vi "Image Flatfield Correction (SGL).vi"(8 "error in (no error)":errorcluster, 10 "Flatfield Correction":T2={"Flatfield Estimation Options"={"Sampling Grid Size X"=0, "Sampling Grid Size Y"=256, "Polynomial Degree"=0}, "Background Options"={"Estimate Background"=FALSE, "Background Estimation Size"=0, "Niblack Deviation Factor [0. 1]"=0.0}, "Correction Factor"=0.0}, 11 "Refnum in":T1) -> (0 "error out":errorcluster, 3 "Refnum out":T1)   [LabVIEW 2021, in "Image.lvlib"]
uses:
  Image.lvlib
  Flatfield Correction Options.ctl
  <vilib>/vision/Image Controls.llb/IMAQ Image.ctl
  <vilib>/vision/Process.llb/Surface Fit Options.ctl
  <vilib>/vision/Process.llb/Background Estimation Options.ctl
  <vilib>/vision/NI_Vision_Development_Module.lvlib
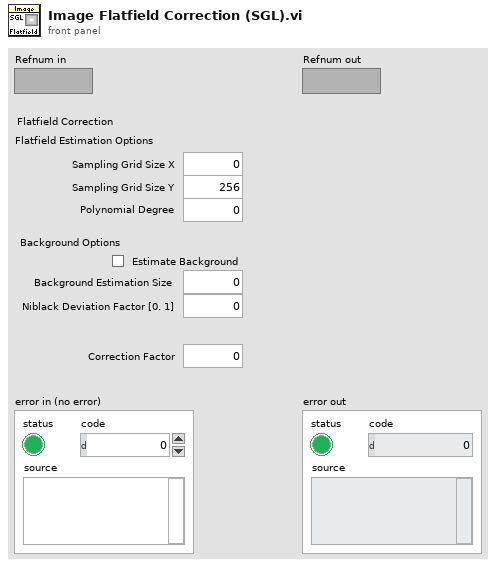
[diagram p1: front panel]
types:
  T1 = typedef "IMAQ Image.ctl" = refnum<image>
  T2 = typedef "Image.lvlib/Flatfield Correction Options.ctl" = cluster{"Flatfield Estimation Options":cluster{"Sampling Grid Size X":i32, "Sampling Grid Size Y":i32, "Polynomial Degree":i32}, "Background Options":cluster{"Estimate Background":bool, "Background Estimation Size":i32, "Niblack Deviation Factor [0. 1]":dbl}, "Correction Factor":sgl}
  T3 = typedef "Background Estimation Options.ctl" = cluster{"Estimate Background?":bool, "Method":i32, "Polynomial Degree":i32, "Window Size (32x32)":cluster{"SizeX":i32, "SizeY":i32}, "Niblack Deviation Factor (0.2)":dbl}
  T4 = cluster{"Line Scan Image?":bool, "Correction Factor":sgl}
  T5 = typedef "Surface Fit Options.ctl" = cluster{"Model":i32, "Sampling Grid Size":cluster{"SizeX":i32, "SizeY":i32}, "Polynomial Degree":i32}
  T6 = typedef "Image Type" = u32
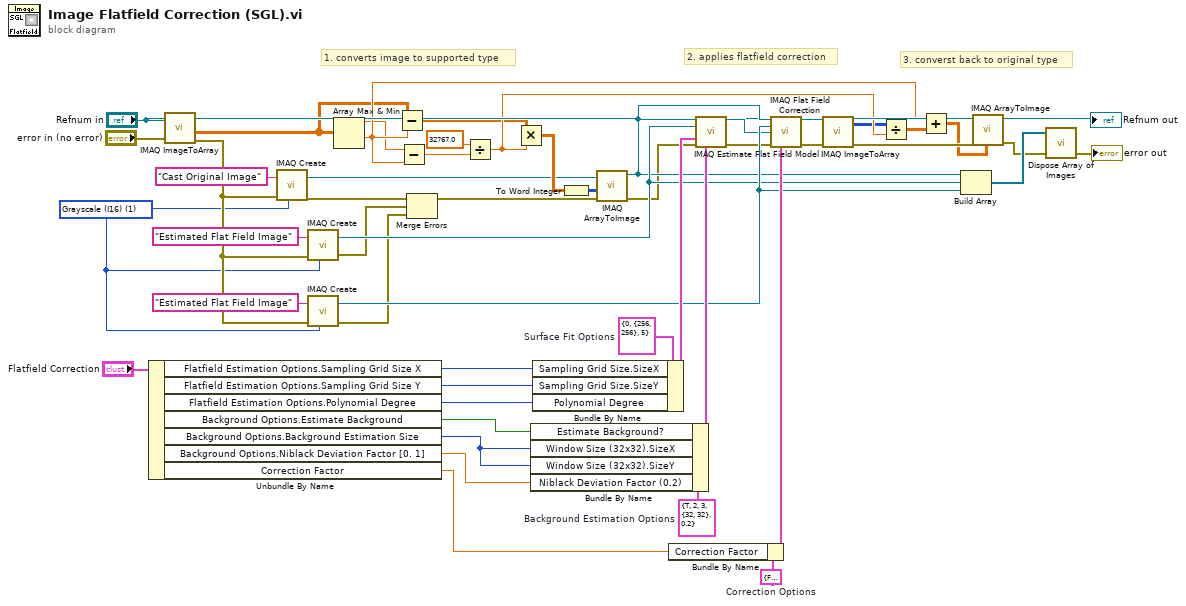
[diagram p0: block diagram]
diagram:
  w51 = T3 {"Estimate Background?"=TRUE, "Method"=2, "Polynomial Degree"=3, "Window Size (32x32)"={"SizeX"=32, "SizeY"=32}, "Niblack Deviation Factor (0.2)"=0.2}  # Background Estimation Options
  w47 = T4 {"Line Scan Image?"=FALSE, "Correction Factor"=1.1}  # Correction Options
  w43 = T5 {"Model"=0, "Sampling Grid Size"={"SizeX"=256, "SizeY"=256}, "Polynomial Degree"=5}  # Surface Fit Options
  w1 = T6 1 items=["Grayscale (U8)", "Grayscale (I16)", "Grayscale (SGL)", "Complex (CSG)", "RGB (U32)", "HSL (U32)", "RGB (U64)", "Grayscale (U16)"] ("New Image Type")
  # "3. converst back to original type"
  # "2. applies flatfield correction"
  # "1. converts image to supported type"
  n1 = Unbundle By Name("Flatfield Correction") -> ("Flatfield Estimation Options.Sampling Grid Size X"=w41:i32, "Flatfield Estimation Options.Sampling Grid Size Y"=w2:i32, "Flatfield Estimation Options.Polynomial Degree"=w42:i32, "Background Options.Estimate Background"=w45:bool, "Background Options.Background Estimation Size"=w48:i32, "Background Options.Niblack Deviation Factor [0. 1]"=w49:dbl, "Correction Factor"=w50:sgl)
  n2 = call "IMAQ ImageToArray"("error in (no error)"="error in (no error)", "Image"="Refnum in") -> ("Image Pixels (Float)"=w7:sgl[][], "error out"=w3:errorcluster)  [unwired: 2 in, 3 out]
  n3 = call "IMAQ Create"("Image Name"="Cast Original Image", "Image Type"=w1, "error in (no error)"=w3) -> ("New Image"=w10:T1, "error out"=w5:errorcluster)  [unwired: 2 in]
  n4 = call "IMAQ Create"("Image Name"="Estimated Flat Field Image", "Image Type"=w1, "error in (no error)"=w3) -> ("New Image"=w36:T1, "error out"=w31:errorcluster)  [unwired: 2 in]
  n5 = call "IMAQ Create"("Image Name"="Estimated Flat Field Image", "Image Type"=w1, "error in (no error)"=w3) -> ("New Image"=w37:T1, "error out"=w34:errorcluster)  [unwired: 2 in]
  n6 = Array Max & Min(array=w7) -> (max value=w8:sgl, min value=w20:sgl)  [unwired: 2 out]
  n7 = Subtract(x=w7, y=w20) -> (x-y=w9:sgl[][])
  n8 = Subtract(x=w8, y=w20) -> (x-y=w16:sgl)
  n9 = Merge Errors(w5, w31, w34) -> (w30:errorcluster)
  n10 = Divide(x=sgl 32767.0, y=w16) -> (x/y=w18:sgl)
  n11 = Multiply(x=w9, y=w18) -> (x*y=w11:sgl[][])
  n12 = Bundle By Name(cluster=w51, "Estimate Background?"=w45, "Window Size (32x32).SizeX"=w48, "Window Size (32x32).SizeY"=w48, "Niblack Deviation Factor (0.2)"=w49) -> (w44:T3)
  n13 = Bundle By Name(cluster=w43, "Sampling Grid Size.SizeX"=w41, "Sampling Grid Size.SizeY"=w2, "Polynomial Degree"=w42) -> (w40:T5)
  n14 = To Word Integer(number=w11) -> (16bit integer=w13:i16[][])
  n15 = call "IMAQ ArrayToImage"("error in (no error)"=w30, "Image Pixels (I16)"=w13, "Image"=w10) -> ("error out"=w12:errorcluster, "Image Out"=w35:T1)  [unwired: 7 in]
  n16 = Bundle By Name(cluster=w47, "Correction Factor"=w50) -> (w46:T4)
  n17 = call "IMAQ Estimate Flat Field Model"("Image Src"=w35, "Image Dst"=w36, "Surface Fit Options"=w40, "error in (no error)"=w12, "Background Estimation Options"=w44) -> ("Flat Field Image Out"=w28:T1, "error out"=w4:errorcluster)  [unwired: 9 in]
  n18 = call "IMAQ Flat Field Correction"("Image Src"=w35, "Image Dst"=w37, "Flat Field Image"=w28, "error in (no error)"=w4, "Correction Options"=w46) -> ("Corrected Image"=w27:T1, "error out"=w14:errorcluster)  [unwired: 8 in, 1 out]
  n19 = call "IMAQ ImageToArray"("error in (no error)"=w14, "Image"=w27) -> ("error out"=w22:errorcluster, "Image Pixels (I16)"=w15:i16[][])  [unwired: 2 in, 3 out]
  n20 = Divide(x=w15, y=w18) -> (x/y=w19:sgl[][])
  n21 = Add(x=w20, y=w19) -> (x+y=w21:sgl[][])
  n22 = Build Array(w35, w36, w37) -> (w38:T1[])
  n23 = call "IMAQ ArrayToImage"("Image Pixels (Float)"=w21, "error in (no error)"=w22, "Image"="Refnum in") -> ("error out"=w25:errorcluster, "Image Out"=→"Refnum out":T1)  [unwired: 7 in]
  n24 = call "Dispose Array of Images.vi"("Array of Images"=w38, "error in (no error)"=w25) -> ("error out"=→"error out":errorcluster)  [unwired: 7 in]
